vi "sm.main.vi"   [LabVIEW 2019]
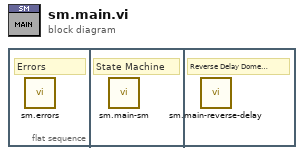
[diagram p0: block diagram]
diagram:
  n1 = flat-sequence {
    frame #0 {
      # "Errors"
      n2 = call "sm.errors.vi"() -> ()  [unwired: 12 in]
    }
    frame #1 {
      # "State Machine"
      n3 = call "sm.main-sm.vi"() -> ()  [unwired: 12 in]
    }
    frame #2 {
      # "Reverse Delay Dome Command"
      n4 = call "sm.main-reverse-delay.vi"() -> ()  [unwired: 12 in]
    }
  }
